vi "proceso3.vi"() -> ()   [LabVIEW 2020]
panel:
  out "proceso 3":T1
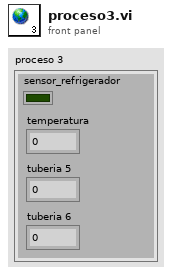
[diagram p1: front panel]
types:
  T1 = cluster{"sensor_refrigerador":bool, "temperatura":dbl, "tuberia 5":u8, "tuberia 6":u8}
diagram:
